vi "get index definition.vi"(10 "channel classification":T1, 11 "Temperature Controller Logic configuration in":refnum<class "Temperature Controller Logic configuration.lvclass">) -> (1 "valid?":bool, 2 "index cluster":variant, 3 "Temperature Controller Logic configuration out":refnum<class "Temperature Controller Logic configuration.lvclass">)   [LabVIEW 2015, in "Temperature Controller Logic configuration.lvclass"]
uses:
  Temperature Controller Logic configuration.lvclass
  <vilib>/NI/Tag Bus Module Framework/channel/channel classification.ctl
  parameter data indices.ctl
  result data indices.ctl
  <vilib>/NI/Tag Bus Module Framework/channel/TBM channel.lvclass
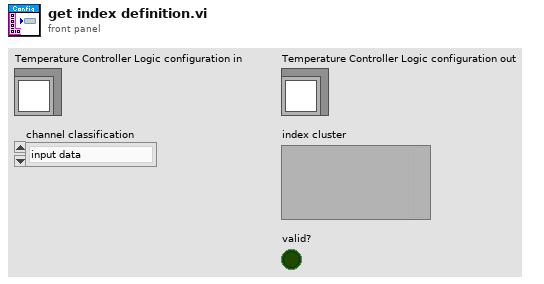
[diagram p1: front panel]
types:
  T1 = typedef "TBM channel.lvclass/channel classification.ctl" = enum16{"input data", "output data", "processing parameter", "processing result"}
  T2 = typedef "Temperature Controller Logic configuration.lvclass/parameter data indices.ctl" = cluster{"Double.Temperature":i32, "Double.setpoint":i32, "Double.output range high":i32, "Double.output range low":i32, "Double.Kc":i32, "Double.Ti":i32, "Double.Td":i32, "Boolean.Fan on?":i32}
  T3 = typedef "Temperature Controller Logic configuration.lvclass/result data indices.ctl" = cluster{"Double.fan":i32, "Double.lamp":i32}
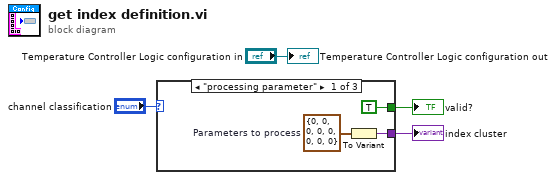
[diagram p0: block diagram]
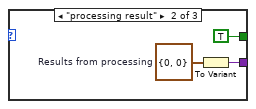
[diagram p2: hidden frame]
diagram:
  n1 = case shown="\"processing parameter\"" "channel classification" {
    tunnel: [TRUE TRUE _] -> w2
    tunnel: [w6 w9 _] -> w1
    frame "processing parameter" {
      w5 = T2 {"Double.Temperature"=0, "Double.setpoint"=0, "Double.output range high"=0, "Double.output range low"=0, "Double.Kc"=0, "Double.Ti"=0, "Double.Td"=0, "Boolean.Fan on?"=0}  # Parameters to process
      n2 = To Variant(anything=w5) -> (Variant=w6:variant)
    }
    frame "processing result" {
      w8 = T3 {"Double.fan"=0, "Double.lamp"=0}  # Results from processing
      n3 = To Variant(anything=w8) -> (Variant=w9:variant)
    }
    frame Default {
    }
  }
  "valid?" <- w2
  "index cluster" <- w1
  "Temperature Controller Logic configuration out" <- "Temperature Controller Logic configuration in"
